vi "CAN.vi"() -> (0 "error out":errorcluster, 1 "CAN":T1, 2 "FPGA VI Reference Out":refnum<k20>)   [LabVIEW 2021]
uses:
  <vilib>/FPGAPlugInAG/cRIO-9068/niLvFpga_Open_cRIO-9068.vi
  <vilib>/FPGAPlugInAG/cRIO-9068/niLvFpga_Run_cRIO-9068.vi
  <vilib>/xnet/xnet.llb/XNET Create Session (Frame Input Stream).vi
  <vilib>/xnet/xnet.llb/XNET Create Session (Frame Output Stream).vi
  <vilib>/rvi/interface/nirviOpenFPGA/nirviOpenFPGA.xnode
  FPGA Bitfiles/pv-emulators_FPGATarget_emptyFPGA_z5uule7UYNw.lvbitx
  <vilib>/rvi/interface/nirviMethod/nirviMethod.xnode
  <resource>/objmgr/xnet.rc
panel:
  out "Devices":refnum<k21>[](array[refnum])
  out "iteration":i32
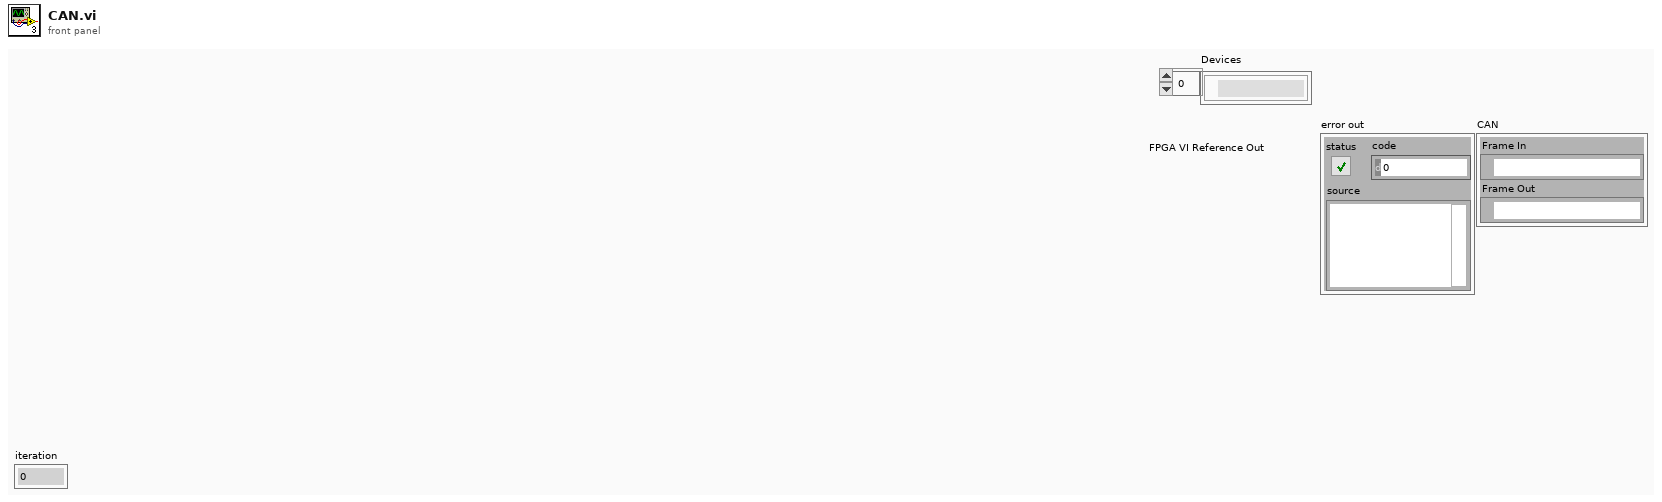
[diagram p1: front panel]
types:
  T1 = cluster{"Frame In":refnum<k21>, "Frame Out":refnum<k21>}
  T2 = cluster{"session out":refnum<k21>, "session out":refnum<k21>}
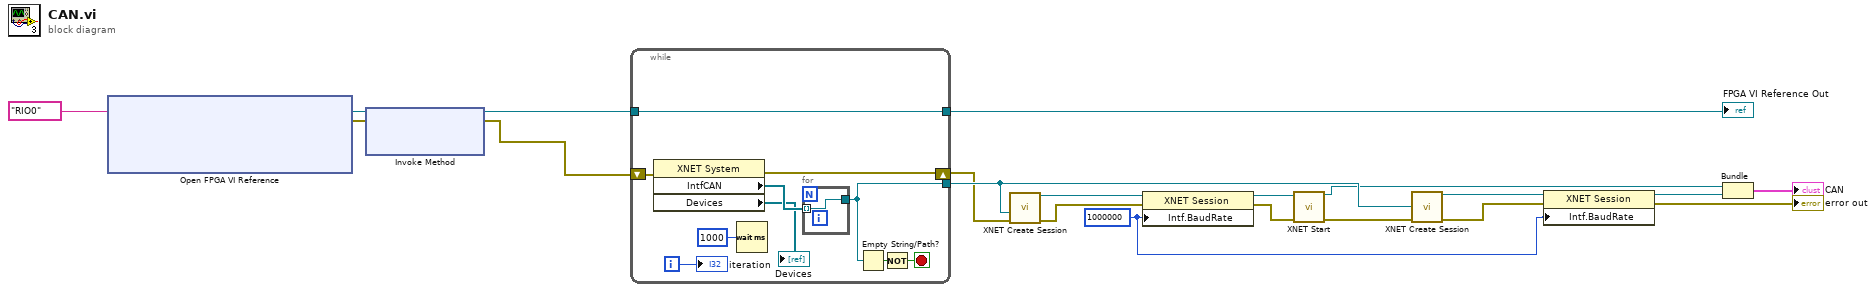
[diagram p0: block diagram]
diagram:
  w13 = u32 1000000 ("y")
  n1 = xnode "Open FPGA VI Reference"("resource name"=tag "RIO0") -> ("FPGA VI Reference Out"=w4:refnum<k20>, "error out"=w6:errorcluster)  [unwired: 1 in]
  n2 = xnode "Invoke Method"("FPGA VI Reference In"=w4, "error in"=w6) -> ("FPGA VI Reference Out"=w3:refnum<k20>, "error out"=w2:errorcluster)  [unwired: 1 in]
  n3 = while {
    tunnel: [w26] -> w12
    tunnel: [w23] -> w7
    tunnel: w3 -> [w23]
    shift-right: [w21] -> w1
    shift-left: w2 -> [w22]
    i -> [w27]
    stop <- w28 stop-if-true
    n4 = property class="XNET System"(error in=w22) -> (error out=w21:errorcluster, "IntfCAN"=w25:refnum<k21>[], "Devices"=→"Devices":refnum<k21>[])  [unwired: 1 in, 1 out]
    n5 = Wait (ms)(milliseconds to wait=u32 1000) -> ()  [unwired: 1 out]
    n6 = for {
      tunnel: w25 -> [w31] mode=indexing
      tunnel: [w31] -> w26
    }
    n7 = Empty String/Path?(string/path=w26) -> (empty?=w29:bool)
    n8 = Not(x=w29) -> (.not. x?=w28:bool)
    "iteration" <- w27
  }
  "FPGA VI Reference Out" <- w7
  n9 = call-poly <vilib>:"XNET Create Session.vi"("interface"=w12, "error in (no error)"=w1) -> ("session out"=w18:refnum<k21>, "error out"=w19:errorcluster)  [unwired: 1 in, 11 out]
  n10 = property class="XNET Session"(reference=w18, error in=w19, "Intf.BaudRate"=w13) -> (reference out=w17:refnum<k21>, error out=w16:errorcluster)
  n11 = call <vilib>:"XNET Start.vi"("session in"=w17, "error in (no error)"=w16) -> ("session out"=w10:refnum<k21>, "error out"=w15:errorcluster)  [unwired: 12 out]
  n12 = call-poly <vilib>:"XNET Create Session.vi"("interface"=w12, "error in (no error)"=w15) -> ("session out"=w20:refnum<k21>, "error out"=w14:errorcluster)  [unwired: 1 in, 11 out]
  n13 = property class="XNET Session"(reference=w20, error in=w14, "Intf.BaudRate"=w13) -> (reference out=w9:refnum<k21>, error out=→"error out":errorcluster)
  n14 = Bundle("session out"=w10, "session out"=w9) -> (→"CAN":T2)  [unwired: 1 in]
